vi "Init.vi"(8 "error in (no error)":errorcluster) -> (0 "error out":errorcluster)   [LabVIEW 2013, in "Advanced Plotting Toolkit.lvlib"]
doc: "Optional VI which manually starts the plotting system. This allows you to put the (1-5 second) startup delay in another thread, or detect (rare) startup errors before calling the plotting VIs."
uses:
  Advanced Plotting Toolkit.lvlib
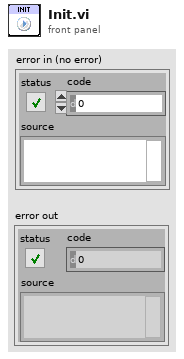
[diagram p1: front panel]
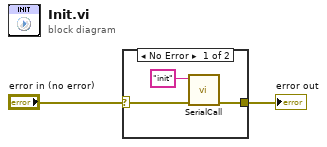
[diagram p0: block diagram]
diagram:
  n1 = case shown="No Error" "error in (no error)" {
    selector: "error in (no error)" -> [w4 w6]
    tunnel: [w3 w6] -> w2
    frame No Error {
      n2 = call "SerialCall.vi"("error in (no error)"=w4, "Resource"="init") -> ("error out"=w3:errorcluster)  [unwired: 8 in, 1 out]
    }
    frame Error {
    }
  }
  "error out" <- w2
